vi "DC Bus Test_TS_BB_v2.vi"(8 "error in (no error)":errorcluster, 10 "HMP4040 VISA":refnum<visa-resource-name>, 11 "Control Board VISA":refnum<visa-resource-name>) -> (0 "error out":errorcluster, 3 "Inv_DC":dbl[](array[numeric]))   [LabVIEW 2022 SP3]
uses:
  ADCSelector BB.ctl
  HMP4040_ChannelControlAutomatic.ctl
panel:
  out "INV B (0V)":dbl
  out "INV A (10V)":dbl
  out "INV B (10V)":dbl
  out "INV A (0V)":dbl
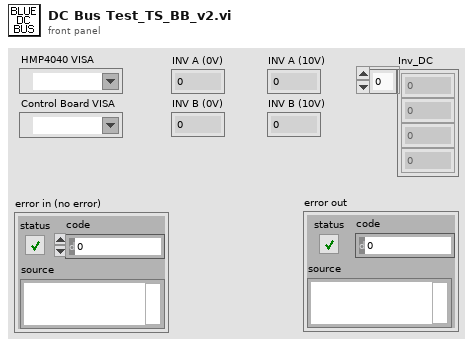
[diagram p1: front panel]
types:
  T1 = typedef "HMP4040_ChannelControlAutomatic.ctl" = enum16{"Off", "Control Power", "HMP2020 Control + DC32V", "HMP2020 Control + DC8V", "HMP4040 Control + DC32V", "HMP4040 Control +DC8V", "HMP4040 Ch2 24V 4A"}
  T2 = typedef "ADCSelector BB.ctl" = enum16{"INVA_ISENSE_U", "INVA_ISENSE_V", "INVA_ISENSE_W", "INVA_UDC", "INVA_TEMP", "HB_TEMP", "AUXB_TEMP", "VLINE_AB", "VLINE_BC", "VLINE_CA", "VSENSE_POS_24V", "VSENSE_POS_5V", "VSENSE_NEG_15V", "INVB_ISENSE_U", "INV_B_ISENSEV", "INVB_ISENSE_W", "INVB_UDC", "INVB_TEMP", "AUXA_TEMP", "AUXC_TEMP", "VOUT_AB", "VOUT_BC", "VOUT_CA", "VSENSE_POS_15V", "VSENSE_POS_3P3V", "TEST_POINT"}
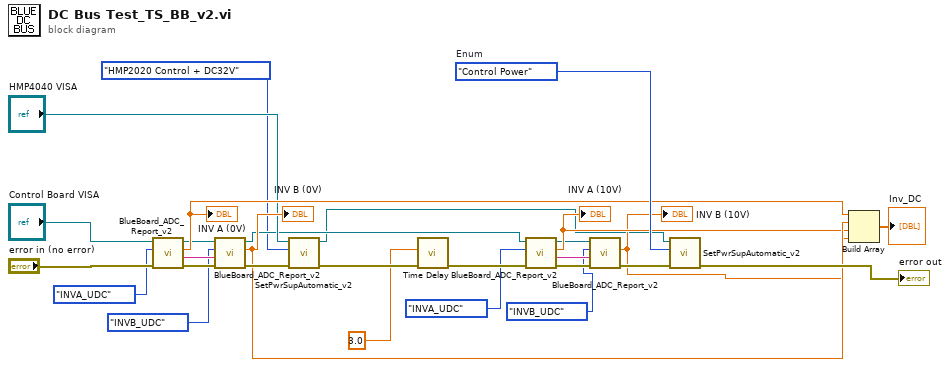
[diagram p0: block diagram]
diagram:
  w16 = HMP4040_ChannelControlAutomatic."Control Power"  # Enum
  n1 = call "BlueBoard_ADC_Report_v2.vi"("error in (no error)"="error in (no error)", "Blue Board Enum"=ADCSelector_BB."INVA_UDC", "ControlBoard VISA"="Control Board VISA") -> ("error out"=w27:errorcluster, "Message OUT"=w26:string, "Result"=w15:dbl, "VISA Refnum out"=w8:refnum<visa-resource-name>)  [unwired: 5 in]
  "INV A (0V)" <- w15
  n2 = call "BlueBoard_ADC_Report_v2.vi"("error in (no error)"=w27, "Message IN"=w26, "Blue Board Enum"=ADCSelector_BB."INVB_UDC", "ControlBoard VISA"=w8) -> ("error out"=w25:errorcluster, "Result"=w14:dbl, "VISA Refnum out"=w7:refnum<visa-resource-name>)  [unwired: 4 in, 1 out]
  "INV B (0V)" <- w14
  n3 = call "SetPwrSupAutomatic_v2.vi"("error in (no error)"=w25, "Enum"=HMP4040_ChannelControlAutomatic."HMP2020 Control + DC32V", "HMP VISA"="HMP4040 VISA") -> ("error out"=w28:errorcluster, "HMP VISA Out"=w1:refnum<visa-resource-name>)  [unwired: 7 in]
  n4 = call "Time Delay"("error in (no error)"=w28, "Delay Time (s)"=3.0) -> ("error out"=w22:errorcluster)  [unwired: 9 in]
  n5 = call "BlueBoard_ADC_Report_v2.vi"("error in (no error)"=w22, "Blue Board Enum"=ADCSelector_BB."INVA_UDC", "ControlBoard VISA"=w7) -> ("error out"=w24:errorcluster, "Message OUT"=w23:string, "Result"=w13:dbl, "VISA Refnum out"=w6:refnum<visa-resource-name>)  [unwired: 5 in]
  "INV A (10V)" <- w13
  n6 = call "BlueBoard_ADC_Report_v2.vi"("error in (no error)"=w24, "Message IN"=w23, "Blue Board Enum"=ADCSelector_BB."INVB_UDC", "ControlBoard VISA"=w6) -> ("error out"=w20:errorcluster, "Result"=w12:dbl)  [unwired: 4 in, 2 out]
  "INV B (10V)" <- w12
  n7 = call "SetPwrSupAutomatic_v2.vi"("error in (no error)"=w20, "Enum"=w16, "HMP VISA"=w1) -> ("error out"=→"error out":errorcluster)  [unwired: 7 in, 1 out]
  n8 = Build Array(w15, w14, w13, w12) -> (→"Inv_DC":dbl[])
